vi "Read FGV DataOut.vi"(7 "TSt/FConveyor":bool, 8 "error in (no error)":errorcluster, 10 "Data":T1, 11 "Vision AI in":refnum<class "Vision AI.lvclass">) -> (0 "error out":errorcluster, 2 "DataOut":string, 3 "Vision AI out":refnum<class "Vision AI.lvclass">)   [LabVIEW 2019, in "Vision AI.lvclass"]
uses:
  Vision AI.lvclass
  Ctrl/Auto Inspection Data Name.ctl
  Ctrl/Auto Inspection Station Name2.ctl
  FlowIOCtrl.lvclass
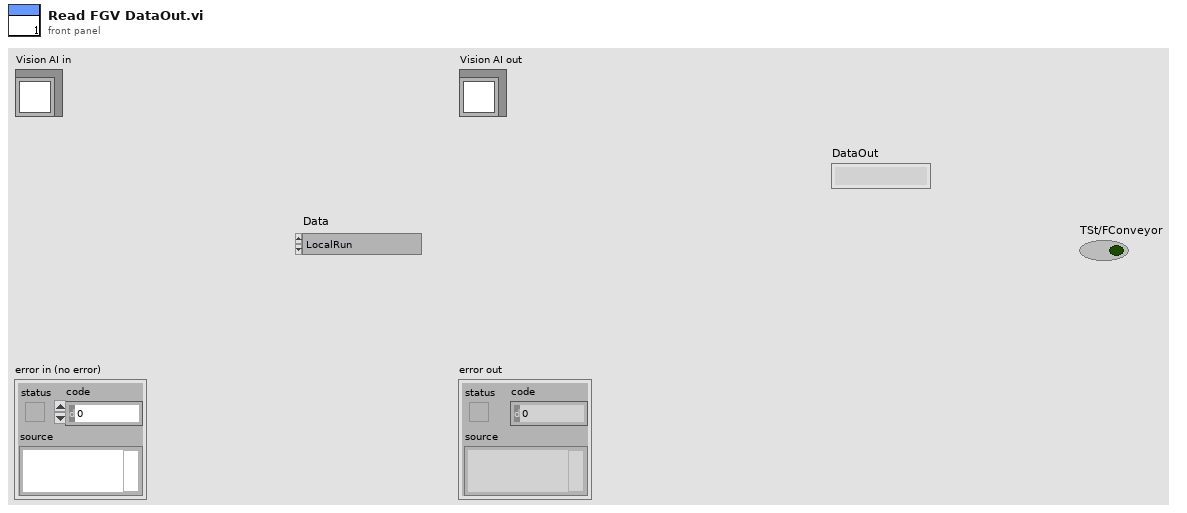
[diagram p1: front panel]
types:
  T1 = typedef "Auto Inspection Data Name.ctl" = enum16{"LocalRun", "ItemSN(TimeCode)", "CurrentAction", "Error", "Data", "OKNG", "電壓值", "電壓值判斷", "電流值", "電流值判斷", "Laser1 Data", "Laser2 Data", "Laser OKNG", "StationNO"}
  T2 = typedef "Auto Inspection Station Name2.ctl" = enum16{"S1Barcode", "S2Measure", "S3Measure", "S4Measure", "S5Measure", "S11_LaserCheck", "S8_Vision AI"}
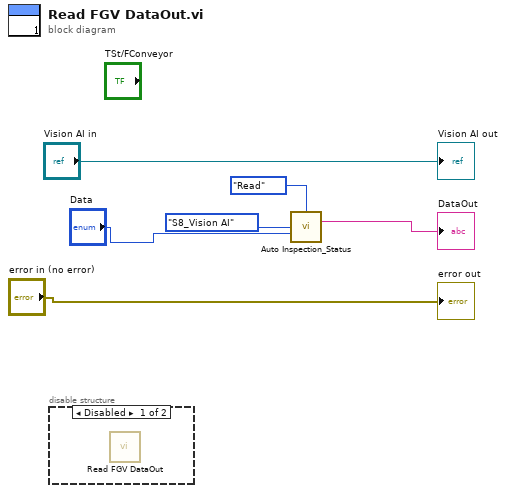
[diagram p0: block diagram]
diagram:
  n1 = disable-structure shown="Disabled" {
    frame Disabled {
      n2 = call-parent "Read FGV DataOut.vi"() -> ()  [unwired: 9 in, 3 out]
    }
    frame Enabled {
    }
  }
  n3 = call "Auto Inspection_Status.vi"("Action"=enum16{"Initial", "Write", "Read"}."Read", "Station"=Auto_Inspection_Station_Name2."S8_Vision AI", "Data"="Data") -> ("DataOut"=→"DataOut":string)  [unwired: 10 in, 2 out]
  "error out" <- "error in (no error)"
  "Vision AI out" <- "Vision AI in"
